vi "Oclaro_FB_INJ_RandomSampling.vi"(1 "Resistance (k Ohms)":dbl=10.0) -> ()   [LabVIEW 2014]
doc: "Use this template to measure or generate signals using the DAQ Assistant Express VI and NI-DAQmx. Double click the DAQ Assistant Express VI to launch a configuration wizard which steps you through configuring a measurement or generation.\n\nNote: You must have an NI-DAQmx compatible device installed to use this Express VI. Refer to the DAQ Quick Start Guide for NI-DAQ 7.0 for a list of compatible devices."
uses:
  Instance           8 18Saved   INJ FB Map .vi
  <instrlib>/Tektronix 7000 Series/Public/Data/Read (Single Waveform).vi
  <instrlib>/Tektronix 7000 Series/Tektronix 7000 Series.lvlib
  <userlib>/libbristoldlv/libbristoldlv.lvlib
  <userlib>/libbristoldlv/libbristoldlv.dll
panel:
  in  "Reset to 0 between settings?":bool
  out "Current Source":string="PROFILE-ITC510"
  out "Total Time (hrs)":dbl=23.33940424164136
  out "Finish time":timestamp=timestamp(3525397732.18738 s since 1904-01-01)
  out "Current INJ":dbl
  in  "file path":path=path "Z:/Toomey/Experimental Data/Oclaro/2015-09-18/Run01/Data"
  in  "Time Series Length":dbl=500000.0
  in  "OSA Model":string="Bristol-771"
  in  "Scope Model":string="Tektronix MSO 71254"
  in  "Exit":bool
  out "Iteration":i32
  out "Spectral Peak":dbl=0.8513913993644499 format="%#_10g"
  in  "Units":enum16{"GHz", "um", "cm-1"}(ring)=enum."um"
  in  "Max Wavelength (um)":ext=0.9
  in  "Min Wavelength (um)":ext=0.8
  out "Instrument Status:":string="OK"
  out "temperature":dbl=29.80661392211914
  out "pressure":dbl=779.7882080078125
  in  "Model":bool=TRUE
  in  "Channel (0: Channel 1)":u16(ring)=3 format="%#_5f" items=["Channel 1", "Channel 2", "Channel 3", "Channel 4", "Math 1", "Math 2", "Math 3", "Math 4", "Reference 1", "Reference 2", "Reference 3", "Reference 4"]
  out "Current AOM":dbl=0.9
  in  "Network Address":string="10.199.199.1"
  out "CL DLL Version":string="5.4.0"
  out "LV DLL Version":string="5.1.0"
  in  "Resolution":bool=TRUE
  in  "Select Wavelength Range":T1(ring)=enum."NIR II: 633 - 1700 nm"
  out "Error out":errorcluster
  in  "Capture OSA?":bool=TRUE
  in  "AOM Step":dbl=0.005
  in  "AOM Finish":dbl=0.9
  in  "AOM Start":dbl=0.1
  in  "Initial Current (mA)":dbl=15.0
  in  "Step Size (mA)":dbl=0.5
  in  "Max Current (mA)":dbl=85.0
  in  "AOM Channel":bool
  out "Start time":timestamp=timestamp(3523998390.26649 s since 1904-01-01)
  in  "Current Source Address":refnum<visa-resource-name>="GPIB0::3::INSTR"
  in  "TEC Address":refnum<visa-resource-name>="GPIB0::3::INSTR"
  in  "Tek Scope Address":refnum<visa-resource-name>="GPIB0::4::INSTR"
  in  "Time to wait for TEC (sec)":dbl=3.0 caption="Delay Time (s)"
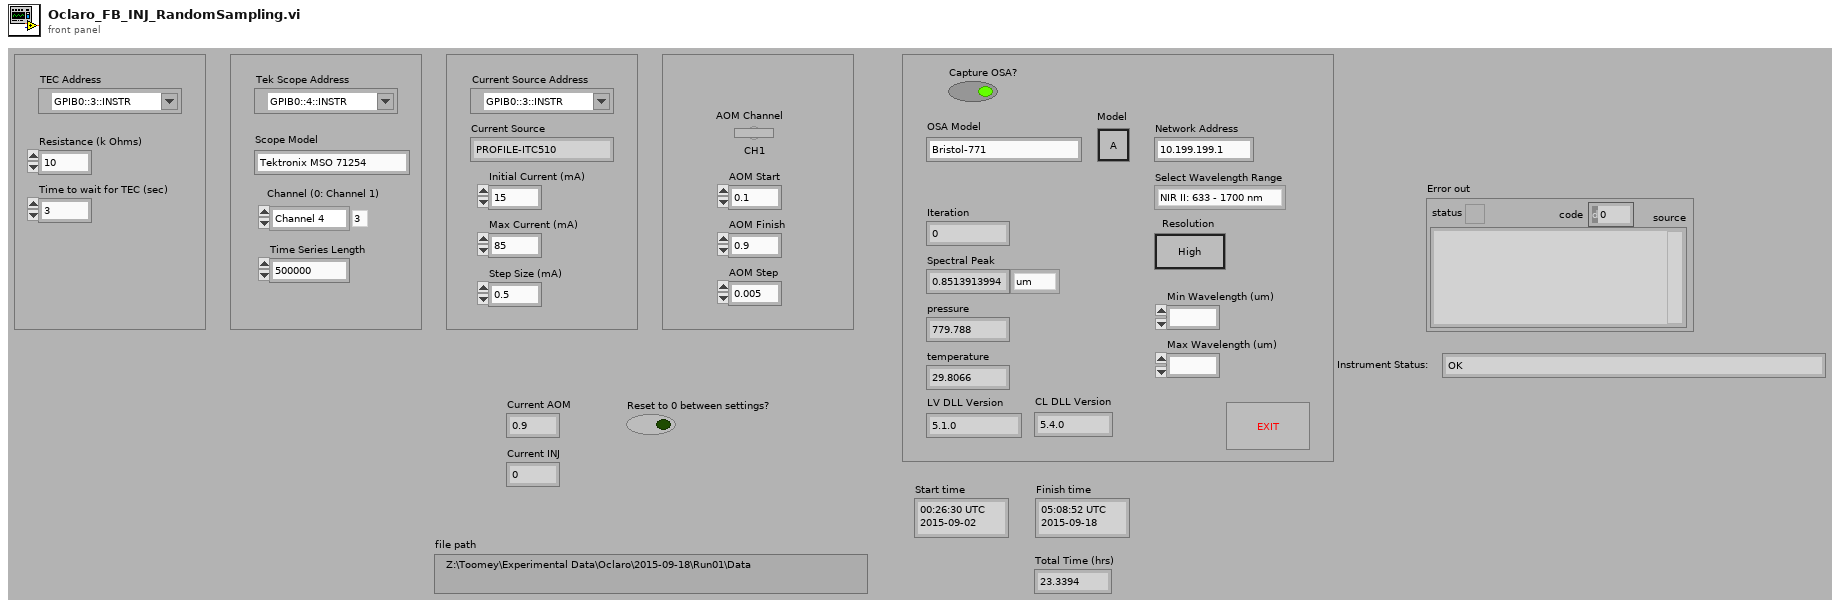
[diagram p1: front panel]
types:
  T1 = enum16{"VIS I: 375 - 633 nm", "VIS II: 633 - 1100 nm", "NIR I: 520 - 633 nm", "NIR II: 633 - 1700 nm", "IR: 1,000 - 5,000 nm", "MIR: 2,000 - 12,000 nm"}
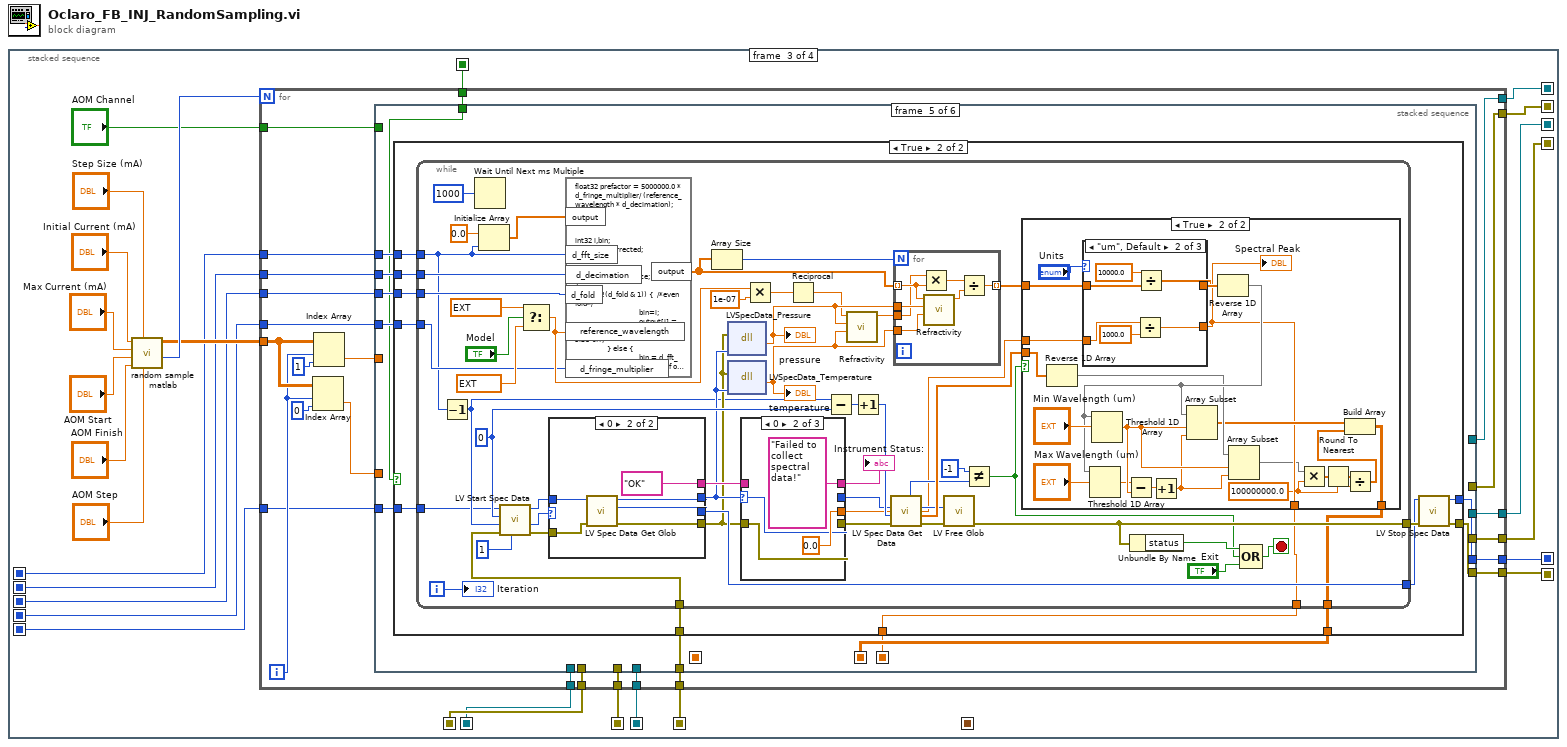
[diagram p0: block diagram]
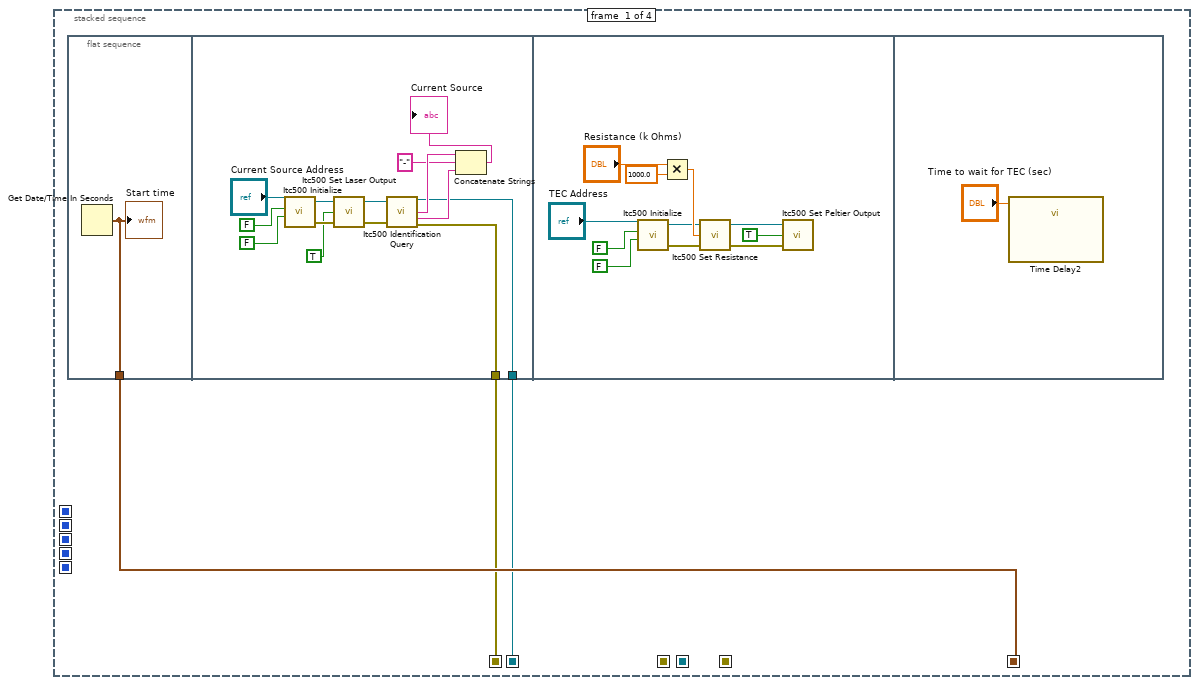
[diagram p2: hidden frame]
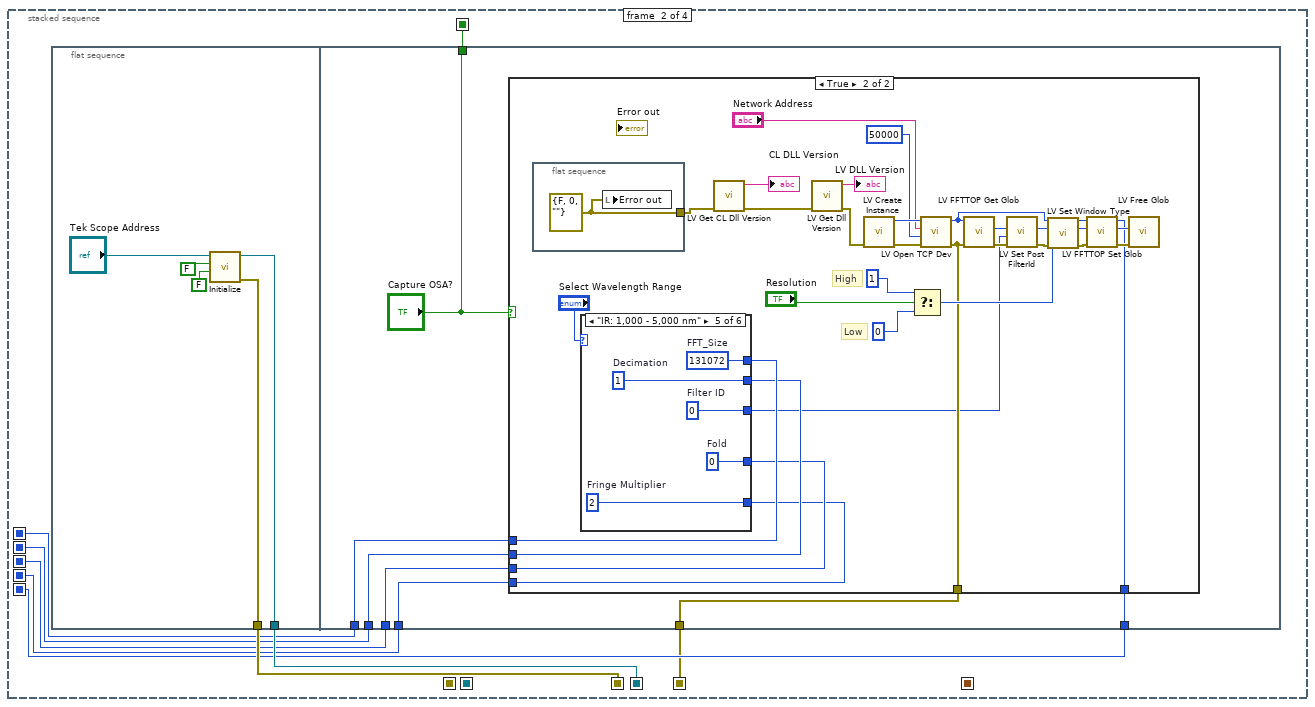
[diagram p3: hidden frame]
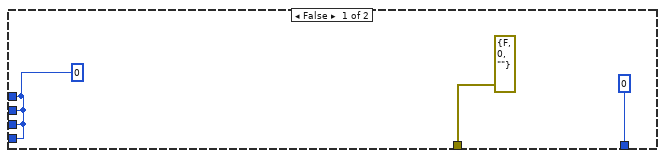
[diagram p4: hidden frame]
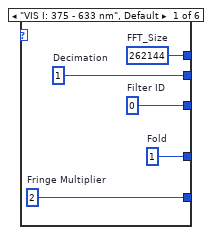
[diagram p5: hidden frame]
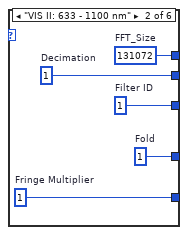
[diagram p6: hidden frame]
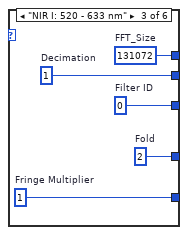
[diagram p7: hidden frame]
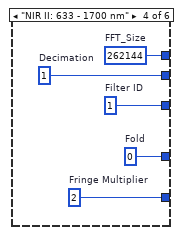
[diagram p8: hidden frame]
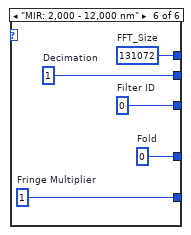
[diagram p9: hidden frame]
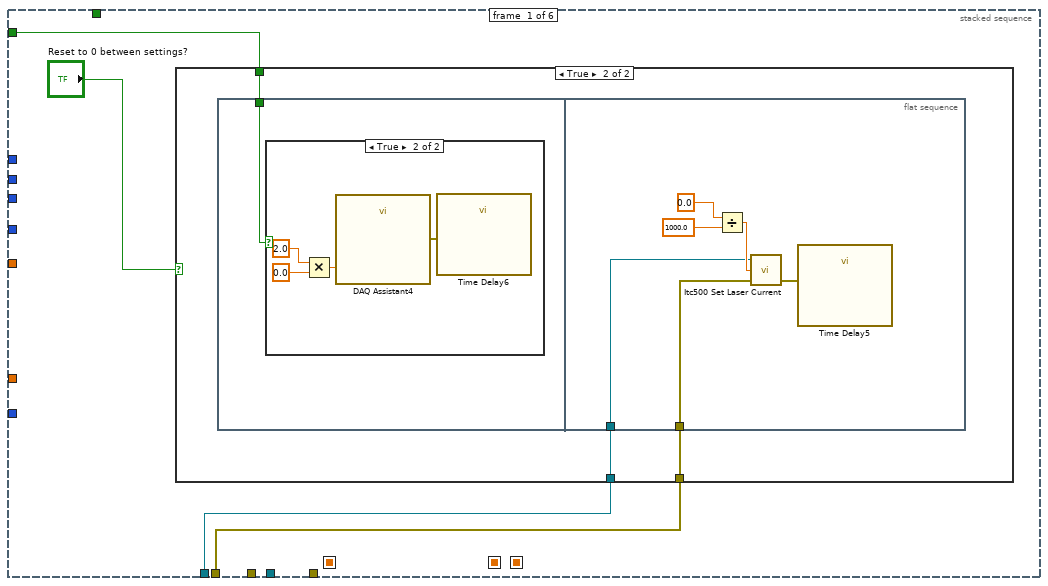
[diagram p10: hidden frame]
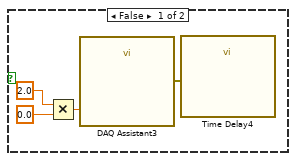
[diagram p12: hidden frame]
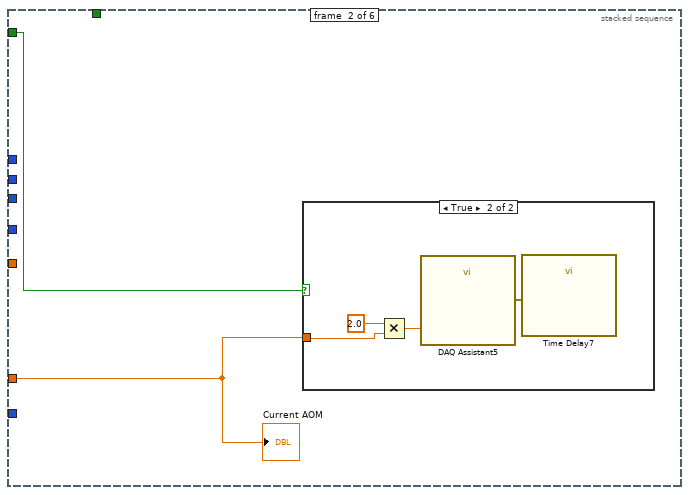
[diagram p13: hidden frame]
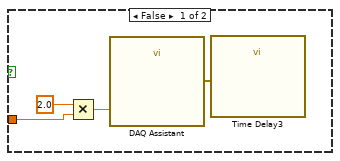
[diagram p14: hidden frame]
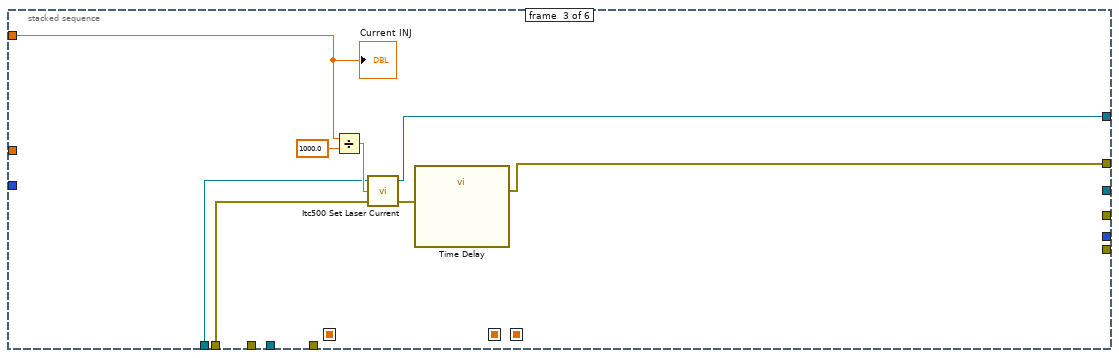
[diagram p15: hidden frame]
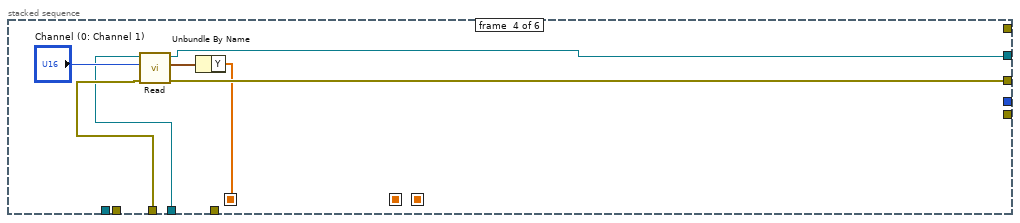
[diagram p16: hidden frame]
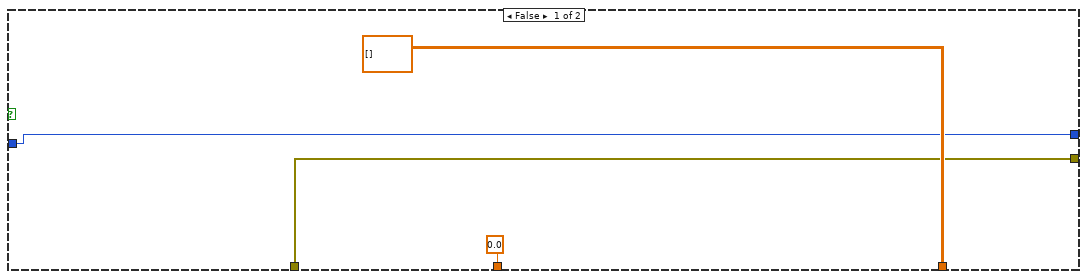
[diagram p17: hidden frame]
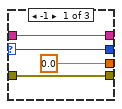
[diagram p18: hidden frame]
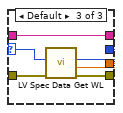
[diagram p19: hidden frame]
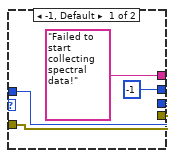
[diagram p20: hidden frame]
diagram:
  n1 = stacked-sequence {
    seq-local: [_ w38 _ _] -> [_ _ w121 _]
    seq-local: [_ w39 _ _] -> [_ _ w120 _]
    seq-local: [_ _ w122 _] -> [_ _ _ w383]
    seq-local: [_ _ w123 _] -> [_ _ _ w382]
    seq-local: [w3 _ _ _] -> [_ _ _ w384]
    seq-local: [_ _ w119 _] -> [_ _ _ w381]
    seq-local: [_ _ w118 _] -> [_ _ _ w380]
    seq-local: [w1 _ _ _] -> [_ _ w133 _]
    seq-local: [w2 _ _ _] -> [_ _ w134 _]
    seq-local: [_ w34 _ _] -> [_ _ w130 _]
    seq-local: [_ w35 _ _] -> [_ _ w129 _]
    seq-local: [_ w36 _ _] -> [_ _ w128 _]
    seq-local: [_ w37 _ _] -> [_ _ w127 _]
    seq-local: [_ w33 _ _] -> [_ _ w126 _]
    seq-local: [_ w32 _ _] -> [_ _ w125 _]
    seq-local: [_ w31 _ _] -> [_ _ w124 _]
    seq-local: [_ _ w117 _] -> [_ _ _ w379]
    seq-local: [_ _ w116 _] -> [_ _ _ w378]
    frame #0 {
      n2 = flat-sequence {
        tunnel: [w4] -> w3
        tunnel: [w7] -> w2
        tunnel: [w5] -> w1
        frame #0 {
          n3 = Get Date/Time In Seconds() -> (seconds since 1Jan1904=w4:timestamp)
          "Start time" <- w4
        }
        frame #1 {
          n4 = call <instrlib>:"Itc500 Initialize.vi"("reset device"=FALSE, "id query"=FALSE, "resource name"="Current Source Address") -> ("error out"=w18:errorcluster, "instrument handle"=w17:refnum<visa-resource-name>)  [unwired: 1 in, 1 out]
          n5 = call <instrlib>:"Itc500 Set Laser Output.vi"("error in (no error)"=w18, "output"=TRUE, "instrument handle"=w17) -> ("error out"=w8:errorcluster, "instrument handle out"=w6:refnum<visa-resource-name>)  [unwired: 1 out]
          n6 = call <instrlib>:"Itc500 Identification Query.vi"("instrument handle"=w6, "error in (no error)"=w8) -> ("instrument handle out"=w5:refnum<visa-resource-name>, "manufacturer name"=w12:string, "instrument name"=w11:string, "error out"=w7:errorcluster)  [unwired: 7 in, 3 out]
          n7 = Concatenate Strings(w12, "-" ("string"), w11) -> (→"Current Source":string)
        }
        frame #2 {
          n8 = call <instrlib>:"Itc500 Initialize.vi"("reset device"=FALSE, "id query"=FALSE, "resource name"="TEC Address") -> ("error out"=w25:errorcluster, "instrument handle"=w24:refnum<visa-resource-name>)  [unwired: 1 in, 1 out]
          n9 = Multiply(x="Resistance (k Ohms)", y=1000.0) -> (x*y=w28:dbl)
          n10 = call <instrlib>:"Itc500 Set Resistance.vi"("error in (no error)"=w25, "resistance"=w28, "instrument handle"=w24) -> ("error out"=w22:errorcluster, "instrument handle out"=w21:refnum<visa-resource-name>)  [unwired: 1 out]
          n11 = call <instrlib>:"Itc500 Set Peltier Output.vi"("error in (no error)"=w22, "output"=TRUE, "instrument handle"=w21) -> ()  [unwired: 3 out]
        }
        frame #3 {
          n12 = call "Time Delay2"("Delay Time (s)"="Time to wait for TEC (sec)") -> ()  [unwired: 10 in, 1 out]
        }
      }
    }
    frame #1 {
      n13 = flat-sequence {
        tunnel: [w41] -> w39
        tunnel: [w40] -> w38
        tunnel: [w51] -> w37
        tunnel: [w50] -> w36
        tunnel: [w49] -> w35
        tunnel: [w48] -> w34
        tunnel: ["Capture OSA?"] -> w33
        tunnel: [w46] -> w32
        tunnel: [w45] -> w31
        frame #0 {
          n14 = call <instrlib>:"Initialize.vi"("Reset? ( Yes)"=FALSE ("Reset (T: Reset)"), "ID Query? ( Yes)"=FALSE ("Reset (T: Reset)"), "VISA resource name"="Tek Scope Address") -> ("error out"=w40:errorcluster, "VISA resource name out"=w41:refnum<visa-resource-name>)  [unwired: 7 in]
        }
        frame #1 {
          n15 = case shown="True" "Capture OSA?" {
            tunnel: [errorcluster {"status"=FALSE, "code"=0, "source"=""} ("error out") w63] -> w45
            tunnel: [0 ("Handle out") w62] -> w46
            tunnel: [w52 w60] -> w48
            tunnel: [w52 w59] -> w49
            tunnel: [w52 w58] -> w50
            tunnel: [w52 w57] -> w51
            frame False {
              w52 = 0 ("FFT_Size")
            }
            frame True {
              # "High"
              # "Low"
              n16 = flat-sequence {
                tunnel: [w84] -> w56
                frame #0 {
                  w84 = errorcluster {"status"=FALSE, "code"=0, "source"=""} ("error out")
                  n17 = local write "Error out"(w84) -> ()
                }
              }
              n18 = case shown="\"IR: 1,000 - 5,000 nm\"" "Select Wavelength Range" {
                tunnel: [w89 w91 w96 w101 w106 w114] -> w57
                tunnel: [w88 w92 w97 w102 w107 w113] -> w58
                tunnel: [w87 w93 w98 w103 w108 w112] -> w59
                tunnel: [w86 w94 w99 w104 w109 w111] -> w60
                tunnel: [w85 w90 w95 w100 w105 w110] -> w55
                frame "VIS I: 375 - 633 nm", Default {
                  w85 = i8 0  # Filter ID
                  w89 = 2  # Fringe Multiplier
                  w88 = 1  # Fold
                  w87 = 1  # Decimation
                  w86 = 262144  # FFT_Size
                }
                frame "VIS II: 633 - 1100 nm" {
                  w90 = i8 1  # Filter ID
                  w91 = 1  # Fringe Multiplier
                  w92 = 1  # Fold
                  w93 = 1  # Decimation
                  w94 = 131072  # FFT_Size
                }
                frame "NIR I: 520 - 633 nm" {
                  w95 = i8 0  # Filter ID
                  w96 = 1  # Fringe Multiplier
                  w97 = 2  # Fold
                  w98 = 1  # Decimation
                  w99 = 131072  # FFT_Size
                }
                frame "NIR II: 633 - 1700 nm" {
                  w100 = i8 1  # Filter ID
                  w101 = 2  # Fringe Multiplier
                  w102 = 0  # Fold
                  w103 = 1  # Decimation
                  w104 = 262144  # FFT_Size
                }
                frame "IR: 1,000 - 5,000 nm" {
                  w105 = i8 0  # Filter ID
                  w106 = 2  # Fringe Multiplier
                  w107 = 0  # Fold
                  w108 = 1  # Decimation
                  w109 = 131072  # FFT_Size
                }
                frame "MIR: 2,000 - 12,000 nm" {
                  w110 = i8 0  # Filter ID
                  w114 = 1  # Fringe Multiplier
                  w113 = 0  # Fold
                  w112 = 1  # Decimation
                  w111 = 131072  # FFT_Size
                }
              }
              n19 = call <userlib>:"LV Get CL Dll Version.vi"("error in (no error)"=w56) -> ("error out"=w76:errorcluster, "str out"=→"CL DLL Version":string)  [unwired: 8 in]
              n20 = call <userlib>:"LV Get Dll Version.vi"("error in (no error)"=w76) -> ("error out"=w77:errorcluster, "str out"=→"LV DLL Version":string)  [unwired: 8 in]
              n21 = call <userlib>:"LV Create Instance.vi"("error in (no error)"=w77) -> ("error out"=w80:errorcluster, "function return (Handle)"=w83:i32)  [unwired: 9 in]
              n22 = Select(t=i8 1, s="Resolution", f=i8 0) -> (s? t:f=w64:i8)
              n23 = call <userlib>:"LV Open TCP Dev.vi"("error in (no error)"=w80, "Port"=u16 50000 ("IP Port"), "TCP/IP Address"="Network Address", "Handle in"=w83) -> ("error out"=w63:errorcluster, "Handle out"=w73:i32)  [unwired: 6 in]
              n24 = call <userlib>:"LV FFTTOP Get Glob.vi"("error in (no error)"=w63, "Handle in"=w73) -> ("error out"=w74:errorcluster, "GHandle out"=w75:i32)  [unwired: 7 in, 1 out]
              n25 = call <userlib>:"LV Set Post FilterId.vi"("error in (no error)"=w74, "Filter ID"=w55, "GHandle in"=w75) -> ("error out"=w69:errorcluster, "GHandle out"=w70:i32)  [unwired: 7 in]
              n26 = call <userlib>:"LV Set Window Type.vi"("error in (no error)"=w69, "Resolution"=w64, "GHandle in"=w70) -> ("error out"=w68:errorcluster)  [unwired: 5 in, 2 out]
              n27 = call <userlib>:"LV FFTTOP Set Glob.vi"("error in (no error)"=w68, "GHandle in"=w70, "Handle in"=w73) -> ("error out"=w71:errorcluster, "GHandle out"=w72:i32, "Handle out"=w62:i32)  [unwired: 6 in]
              n28 = call <userlib>:"LV Free Glob.vi"("error in (no error)"=w71, "GHandle in"=w72) -> ()  [unwired: 9 in, 1 out]
            }
          }
        }
      }
    }
    frame #2 {
      n29 = call "random sample matlab.vi"("AOM delta"="AOM Step", "INJ delta"="Step Size (mA)", "AOM end"="AOM Finish", "AOM start"="AOM Start", "INJ end"="Max Current (mA)", "INJ start"="Initial Current (mA)") -> ("No. of parameters"=w132:i32, "Shuffled Parameters"=w131:dbl[][])  [unwired: 4 in]
      n30 = for {
        N: w132 -> [_]
        tunnel: w134 -> [w164]
        tunnel: w133 -> [w163]
        tunnel: w131 -> [w161]
        tunnel: w130 -> [w156]
        tunnel: w129 -> [w155]
        tunnel: w128 -> [w154]
        tunnel: w127 -> [w153]
        tunnel: w126 -> [w152]
        tunnel: w125 -> [w151]
        tunnel: w124 -> [w150]
        tunnel: [w149] -> w123
        tunnel: [w148] -> w122
        tunnel: w121 -> [w147]
        tunnel: w120 -> [w146]
        tunnel: [w145] -> w119
        tunnel: [w144] -> w118
        tunnel: [w143] -> w117
        tunnel: [w142] -> w116
        tunnel: "AOM Channel" -> [w141]
        i -> [w160]
        n31 = Index Array(array=w161, index (row)=w160, index (col)=0 ("disabled index (col)")) -> (element=w157:dbl)
        n32 = Index Array(array=w161, index (row)=w160, index (col)=1 ("disabled index (col)")) -> (element=w158:dbl)
        n33 = stacked-sequence {
          seq-local: [_ _ _ w207 _ _] -> [_ _ _ _ _ w375]
          seq-local: [_ _ _ _ w222 _] -> [_ _ _ _ _ w364]
          seq-local: [_ _ _ _ w219 _] -> [_ _ _ _ _ w363]
          tunnel: [_ _ w199 _ _ _] -> w149
          tunnel: [_ _ _ w210 _ _] -> w145
          tunnel: [_ _ _ w208 _ _] -> w144
          tunnel: w164 -> [w167 _ w201 _ _ _]
          tunnel: w163 -> [w168 _ w200 _ _ _]
          tunnel: [_ _ w198 _ _ _] -> w148
          tunnel: [_ _ _ _ w221 _] -> w143
          tunnel: [_ _ _ _ w220 _] -> w142
          tunnel: w158 -> [_ _ w197 _ _ _]
          tunnel: w157 -> [_ w188 _ _ _ _]
          tunnel: w156 -> [_ _ _ _ w218 _]
          tunnel: w155 -> [_ _ _ _ w217 _]
          tunnel: w154 -> [_ _ _ _ w216 _]
          tunnel: w153 -> [_ _ _ _ w215 _]
          tunnel: w152 -> [_ _ _ _ w214 w362]
          tunnel: w151 -> [_ _ _ _ w213 _]
          tunnel: w150 -> [_ _ _ _ w212 _]
          tunnel: w147 -> [_ _ _ w206 _ _]
          tunnel: w146 -> [_ _ _ w205 _ _]
          tunnel: w141 -> [w165 w187 _ _ _ _]
          frame #0 {
            n34 = case shown="True" "Reset to 0 between settings?" {
              tunnel: w168 -> [_ w171]
              tunnel: w167 -> [_ w170]
              tunnel: w165 -> [_ w169]
              frame False {
              }
              frame True {
                n35 = flat-sequence {
                  tunnel: w169 -> [w172]
                  tunnel: w171 -> [w183]
                  tunnel: w170 -> [w182]
                  frame #0 {
                    n36 = case shown="True" w172 {
                      frame False {
                        n37 = Multiply(x=2.0, y=0.0 ("data")) -> (x*y=w173:dbl)
                        n38 = call "DAQ Assistant3"("data"=w173) -> ("error out"=w176:errorcluster)  [unwired: 17 in, 1 out]
                        n39 = call "Time Delay4"("error in (no error)"=w176) -> ()  [unwired: 10 in, 1 out]
                      }
                      frame True {
                        n40 = Multiply(x=2.0, y=0.0 ("data")) -> (x*y=w180:dbl)
                        n41 = call "DAQ Assistant4"("data"=w180) -> ("error out"=w177:errorcluster)  [unwired: 17 in, 1 out]
                        n42 = call "Time Delay6"("error in (no error)"=w177) -> ()  [unwired: 10 in, 1 out]
                      }
                    }
                  }
                  frame #1 {
                    n43 = Divide(x=0.0, y=1000.0) -> (x/y=w184:dbl)
                    n44 = call <instrlib>:"Itc500 Set Laser Current.vi"("error in (no error)"=w182, "current"=w184, "instrument handle"=w183) -> ("error out"=w185:errorcluster)  [unwired: 2 out]
                    n45 = call "Time Delay5"("error in (no error)"=w185) -> ()  [unwired: 10 in, 1 out]
                  }
                }
              }
            }
          }
          frame #1 {
            n46 = case shown="True" w187 {
              tunnel: w188 -> [w189 w193]
              frame False {
                n47 = Multiply(x=2.0, y=w189) -> (x*y=w192:dbl)
                n48 = call "DAQ Assistant"("data"=w192) -> ("error out"=w191:errorcluster)  [unwired: 17 in, 1 out]
                n49 = call "Time Delay3"("error in (no error)"=w191) -> ()  [unwired: 10 in, 1 out]
              }
              frame True {
                n50 = Multiply(x=2.0, y=w193) -> (x*y=w194:dbl)
                n51 = call "DAQ Assistant5"("data"=w194) -> ("error out"=w195:errorcluster)  [unwired: 17 in, 1 out]
                n52 = call "Time Delay7"("error in (no error)"=w195) -> ()  [unwired: 10 in, 1 out]
              }
            }
            "Current AOM" <- w188
          }
          frame #2 {
            n53 = Divide(x=w197, y=1000.0) -> (x/y=w202:dbl)
            n54 = call <instrlib>:"Itc500 Set Laser Current.vi"("error in (no error)"=w201, "current"=w202, "instrument handle"=w200) -> ("error out"=w203:errorcluster, "instrument handle out"=w198:refnum<visa-resource-name>)  [unwired: 1 out]
            n55 = call "Time Delay"("error in (no error)"=w203) -> ("error out"=w199:errorcluster)  [unwired: 10 in]
            "Current INJ" <- w197
          }
          frame #3 {
            n56 = call-poly <instrlib>:"Read.vi"("error in (no error)"=w206, "Channel (0: Channel 1)"="Channel (0: Channel 1)", "VISA resource name"=w205) -> ("error out"=w208:errorcluster, "Waveform Data"=w211:waveform(dbl), "VISA resource name out"=w210:refnum<visa-resource-name>)  [unwired: 6 in]
            n57 = Unbundle By Name(w211) -> ("Y"=w207:dbl[])
          }
          frame #4 {
            n58 = case shown="True" w214 {
              tunnel: [ext[][] [] w238] -> w222
              tunnel: [w224 w235] -> w221
              tunnel: [w223 w234] -> w220
              tunnel: [0.0 w233] -> w219
              tunnel: w218 -> [_ w232]
              tunnel: w217 -> [_ w231]
              tunnel: w216 -> [_ w230]
              tunnel: w215 -> [_ w229]
              tunnel: w213 -> [w224 w228]
              tunnel: w212 -> [w223 w227]
              frame False {
              }
              frame True {
                n59 = while {
                  tunnel: [w279] -> w237
                  tunnel: [w274] -> w236
                  tunnel: [w246] -> w238
                  tunnel: [w245] -> w233
                  tunnel: w232 -> [w239]
                  tunnel: w231 -> [w244]
                  tunnel: w230 -> [w243]
                  tunnel: w229 -> [w242]
                  tunnel: w228 -> [w241]
                  tunnel: w227 -> [w240]
                  i -> [w289]
                  stop <- w251 stop-if-true
                  w284 = 0 ("IP Port")
                  n60 = Decrement(x=w239) -> (x-1=w247:i32)
                  n61 = Wait Until Next ms Multiple(millisecond multiple=u32 1000) -> ()  [unwired: 1 out]
                  n62 = Initialize Array(0.0 ("output variable"), w239) -> (w264:dbl[])
                  n63 = call <userlib>:"LV Start Spec Data.vi"("Count"=1 ("IP Port"), "error in (no error)"=w240, "End Bin"=w247, "Start Bin"=w284, "Handle in"=w241) -> ("error out"=w275:errorcluster, "function return code"=w276:i32, "Handle out"=w281:i32)  [unwired: 3 in]
                  n64 = Select(t=ext 632.9914, s="Model", f=ext 632.991) -> (s? t:f=w252:ext)
                  n65 = case shown="0" w276 {
                    tunnel: w281 -> [w314 w320]
                    tunnel: [-1 ("IP Port") w319] -> w269
                    tunnel: [w314 w318] -> w274
                    tunnel: w275 -> [w313 w317]
                    tunnel: [w313 w316] -> w268
                    tunnel: ["Failed to start collecting spectral data!" "OK"] -> w272
                    frame -1, Default {
                    }
                    frame 0 {
                      n66 = call <userlib>:"LV Spec Data Get Glob.vi"("error in (no error)"=w317, "Handle in"=w320) -> ("error out"=w316:errorcluster, "GHandle out"=w319:i32, "Handle out"=w318:i32)  [unwired: 7 in]
                    }
                  }
                  n67 = formula code="float32 prefactor = 5000000.0 * d_fringe_multiplier/ (reference_wavelength * d_decimation);\n\n\n\nint32 i,bin;\nfloat32 uncorrected;\n\n                \nfor(i = 0; i<d_fft_size; i++)\n{\n         if (!(d_fold & 1)) {  /*even fold*/\n                                bin=i;\n                                output[i] = prefactor * (d_fold + bin/(d_fft_size-0));\n                } else {\n                                bin = d_fft_size - i - 1; /*reverse array if odd fold*/\n                                output[i] = prefactor * (d_fold + 1.0 - bin/d_fft_size);\n                }\n                  \n}"("d_fft_size"=w239, "d_decimation"=w244, "d_fold"=w243, "d_fringe_multiplier"=w242, "output"=w264, "reference_wavelength"=w252) -> ("output"=w259:dbl[])
                  n68 = Array Size(array=w259) -> (size(s)=w267:i32)
                  n69 = dll-call lib="C:/Program Files (x86)/National Instruments/LabVIEW 2014/user.lib/libbristoldlv/libbristoldlv.dll" fn="LVSpecData_Pressure"(error in=w268, "ghandle"=w269) -> ("pressure"=w263:dbl)  [unwired: 3 in, 2 out]
                  "pressure" <- w263
                  n70 = dll-call lib="C:/Program Files (x86)/National Instruments/LabVIEW 2014/user.lib/libbristoldlv/libbristoldlv.dll" fn="LVSpecData_Temperature"(error in=w268, "ghandle"=w269) -> ("temperature"=w262:dbl)  [unwired: 3 in, 2 out]
                  "temperature" <- w262
                  n71 = case shown="0" w269 {
                    selector: w269 -> [w299 w303 w308]
                    tunnel: [0.0 ("IP Port") 0.0 ("IP Port") w310] -> w260
                    tunnel: w268 -> [w298 w302 w309]
                    tunnel: [w299 w303 w307] -> w271
                    tunnel: [w298 w302 w306] -> w273
                    tunnel: [w300 "Failed to collect spectral data!" w305] -> w270
                    tunnel: w272 -> [w300 _ w305]
                    frame -1 {
                    }
                    frame 0 {
                    }
                    frame Default {
                      n72 = call <userlib>:"LV Spec Data Get WL.vi"("GHandle in"=w308, "error in (no error)"=w309) -> ("GHandle out"=w307:i32, "Wavelength"=w310:dbl, "error out"=w306:errorcluster)  [unwired: 6 in]
                    }
                  }
                  "Instrument Status:" <- w270
                  n73 = Multiply(x=w252, y=1e-07) -> (x*y=w255:ext)
                  n74 = Reciprocal(x=w255) -> (1/x=w253:ext)
                  n75 = Subtract(x=w247, y=w284) -> (x-y=w283:i32)
                  n76 = call "Refractivity.vi"("Temp"=w262, "Press"=w263, "Wavelength"=w253) -> ("Index [i]"=w266:ext)  [unwired: 8 in]
                  n77 = Increment(x=w283) -> (x+1=w282:i32)
                  n78 = call <userlib>:"LV Spec Data Get Data.vi"("error in (no error)"=w273, "max len"=w282, "GHandle in"=w271) -> ("error out"=w280:errorcluster, "Spectral Data"=w287:sgl[], "GHandle out"=w285:i32, "function return code"=w278:i32)  [unwired: 4 in]
                  n79 = for {
                    N: w267 -> [_]
                    tunnel: w259 -> [w292] mode=indexing
                    tunnel: [w293] -> w261 mode=indexing
                    tunnel: w263 -> [w296]
                    tunnel: w262 -> [w295]
                    tunnel: w266 -> [w291]
                    n80 = Multiply(x=w291, y=w292) -> (x*y=w294:ext)
                    n81 = call "Refractivity.vi"("Temp"=w295, "Press"=w296, "Wavelength"=w292) -> ("Index [i]"=w290:ext)  [unwired: 8 in]
                    n82 = Divide(x=w294, y=w290) -> (x/y=w293:ext)
                  }
                  n83 = call <userlib>:"LV Free Glob.vi"("error in (no error)"=w280, "GHandle in"=w285) -> ("error out"=w279:errorcluster)  [unwired: 9 in]
                  n84 = Not Equal?(x=-1, y=w278) -> (x != y?=w248:bool)
                  n85 = case shown="True" w248 {
                    tunnel: w287 -> [_ w339]
                    tunnel: w261 -> [_ w343]
                    tunnel: w260 -> [_ w341]
                    tunnel: [ext[][] [] w329] -> w246
                    tunnel: [0.0 w328] -> w245
                    frame False {
                    }
                    frame True {
                      w325 = 100000000.0 ("y")
                      n86 = Reverse 1D Array(array=w339) -> (reversed array=w334:sgl[])
                      n87 = case shown="\"um\", Default" "Units" {
                        tunnel: w343 -> [w349 w355 w360]
                        tunnel: [w347 w354 w360] -> w340
                        tunnel: w341 -> [w344 w352 w359]
                        tunnel: [w346 w351 w357] -> w328
                        frame "GHz" {
                          n88 = Divide(x=299792458.0, y=w344) -> (x/y=w346:dbl)
                          n89 = Multiply(x=w349, y=29.9792458) -> (x*y=w347:ext[])
                        }
                        frame "um", Default {
                          n90 = Divide(x=w352, y=1000.0) -> (x/y=w351:dbl)
                          n91 = Divide(x=10000.0, y=w355) -> (x/y=w354:ext[])
                        }
                        frame "cm-1" {
                          n92 = Multiply(x=w359, y=1e-07) -> (x*y=w358:dbl)
                          n93 = Reciprocal(x=w358) -> (1/x=w357:dbl)
                        }
                      }
                      "Spectral Peak" <- w328
                      n94 = Reverse 1D Array(array=w340) -> (reversed array=w336:ext[])
                      n95 = Threshold 1D Array(2:"Max Wavelength (um)", 3:w336) -> (0:w332:ext)  [unwired: 1 in]
                      n96 = Threshold 1D Array(2:"Min Wavelength (um)", 3:w336) -> (0:w335:ext)  [unwired: 1 in]
                      n97 = Subtract(x=w332, y=w335) -> (x-y=w331:ext)
                      n98 = Increment(x=w331) -> (x+1=w330:ext)
                      n99 = Array Subset(array=w336, index=w335, length=w330) -> (w333:ext[])
                      n100 = Array Subset(array=w334, index=w335, length=w330) -> (w324:sgl[])
                      n101 = Multiply(x=w324, y=w325) -> (x*y=w327:dbl[])
                      n102 = Round To Nearest(number=w327) -> (nearest integer value=w326:dbl[])
                      n103 = Divide(x=w326, y=w325) -> (x/y=w323:dbl[])
                      n104 = Build Array(w333, w323) -> (w329:ext[][])
                    }
                  }
                  n105 = Unbundle By Name(w279) -> ("status"=w250:bool)
                  n106 = Compound Arithmetic op=OR(w250, w248, "Exit") -> (w251:bool)
                  "Iteration" <- w289
                }
                n107 = call <userlib>:"LV Stop Spec Data.vi"("error in (no error)"=w237, "Handle in"=w236) -> ("error out"=w234:errorcluster, "Handle out"=w235:i32)  [unwired: 8 in]
              }
            }
          }
          frame #5 {
            n108 = local read "Current AOM"() -> (w366:dbl)
            n109 = local read "Current INJ"() -> (w361:dbl)
            n110 = local read "Current Source"() -> (w369:string)
            n111 = Path To String(path="file path") -> (string=w377:string)
            n112 = Boolean To (0,1)(Boolean=w362) -> (0, 1=w365:i16)
            n113 = Format Into String(format string="%05.2f", w361) -> (resulting string=w373:string)  [unwired: 2 in, 1 out]
            n114 = Format Into String(format string="%05.3f", w366) -> (resulting string=w374:string)  [unwired: 2 in, 1 out]
            n115 = script code="h5create([file_loc '/INJ_' INJval 'mA_AOM_' FBval 'V.h5'],'/TS',[1 TSlength],'ChunkSize',[1 TSlength],'Deflate',5)\n\nh5writeatt([file_loc '/INJ_' INJval 'mA_AOM_' FBval 'V.h5'],'/','var1',inj);\nh5writeatt([file_loc '/INJ_' INJval 'mA_AOM_' FBval 'V.h5'],'/','var1_name','Injection Current (mA)');\nh5writeatt([file_loc '/INJ_' INJval 'mA_AOM_' FBval 'V.h5'],'/','var2',fb);\nh5writeatt([file_loc '/INJ_' INJval 'mA_AOM_' FBval 'V.h5'],'/','var2_name','AOM_Voltage (V)');\nh5writeatt([file_loc '/INJ_' INJval 'mA_AOM_' FBval 'V.h5'],'/','Current_Source',current);\nh5writeatt([file_loc '/INJ_' INJval 'mA_AOM_' FBval 'V.h5'],'/','Temperature','25C');\n\nh5write([file_loc '/INJ_' INJval 'mA_AOM_' FBval 'V.h5'],'/TS',TSdata,[1 1],size(TSdata));\n\nh5writeatt([file_loc '/INJ_' INJval 'mA_AOM_' FBval 'V.h5'],'/TS','Oscilloscope_model',scope);\nh5writeatt([file_loc '/INJ_' INJval 'mA_AOM_' FBval 'V.h5'],'/TS','Sample_interval',20e-12);\nh5writeatt([file_loc '/INJ_' INJval 'mA_AOM_' FBval 'V.h5'],'/TS','Vertical_Scale','10mV/div');\nh5writeatt([file_loc '/INJ_' INJval 'mA_AOM_' FBval 'V.h5'],'/TS','Acquisition_Mode','Sample');\nh5writeatt([file_loc '/INJ_' INJval 'mA_AOM_' FBval 'V.h5'],'/TS','Sampling_Mode','Real-time');\n\nif spec == 1\nsize(OSAdata)\nh5create([file_loc '/INJ_' INJval 'mA_AOM_' FBval 'V.h5'],'/OSA',size(OSAdata),'ChunkSize',[1 length(OSAdata)],'Deflate',5)\nh5write([file_loc '/INJ_' INJval 'mA_AOM_' FBval 'V.h5'],'/OSA',OSAdata,[1 1],size(OSAdata));\nh5writeatt([file_loc '/INJ_' INJval 'mA_AOM_' FBval 'V.h5'],'/OSA','OSA_model',osa);\nh5writeatt([file_loc '/INJ_' INJval 'mA_AOM_' FBval 'V.h5'],'/OSA','Resolution','High');\nh5writeatt([file_loc '/INJ_' INJval 'mA_AOM_' FBval 'V.h5'],'/OSA','Wavelength_Peak',wP);\nend"("file_loc"=w377, "INJval"=w373, "FBval"=w374, "TSlength"="Time Series Length", "TSdata"=w375, "OSAdata"=w364, "inj"=w361, "fb"=w366, "current"=w369, "scope"="Scope Model", "osa"="OSA Model", "spec"=w365, "wP"=w363) -> ()  [unwired: 1 in, 1 out]
          }
        }
      }
    }
    frame #3 {
      n116 = flat-sequence {
        tunnel: w383 -> [w386]
        tunnel: w382 -> [w385]
        tunnel: w381 -> [w393]
        tunnel: w380 -> [w392]
        tunnel: w384 -> [w395]
        tunnel: w379 -> [w411]
        tunnel: w378 -> [w410]
        frame #0 {
          n117 = call <instrlib>:"Itc500 Set Laser Current.vi"("error in (no error)"=w385, "current"=0.0, "instrument handle"=w386) -> ("error out"=w389:errorcluster, "instrument handle out"=w388:refnum<visa-resource-name>)  [unwired: 1 out]
          n118 = call <instrlib>:"Itc500 Set Laser Output.vi"("error in (no error)"=w389, "output"=FALSE, "instrument handle"=w388) -> ()  [unwired: 3 out]
        }
        frame #1 {
          n119 = call "DAQ Assistant2"("data"=0.0) -> ()  [unwired: 17 in, 2 out]
        }
        frame #2 {
          n120 = call <instrlib>:"Close.vi"("error in (no error)"=w392, "VISA resource name"=w393) -> ()  [unwired: 9 in, 1 out]
        }
        frame #3 {
          n121 = Get Date/Time In Seconds() -> (seconds since 1Jan1904=w404:timestamp)
          "Finish time" <- w404
          n122 = local read "file path"() -> (w394:path)
          n123 = Format Date/Time String(seconds (now)=w395) -> (date/time string=w405:string)  [unwired: 2 in]
          n124 = Subtract(x=w404, y=w395) -> (x-y=w408:dbl)
          n125 = Divide(x=w408, y=3600.0) -> (x/y=→"Total Time (hrs)":dbl)
          n126 = Path To String(path=w394) -> (string=w397:string)
          n127 = Concatenate Strings(w397, "\\info.txt" ("string")) -> (w399:string)
          n128 = Format Date/Time String(seconds (now)=w404) -> (date/time string=w401:string)  [unwired: 2 in]
          n129 = String To Path(string=w399) -> (path=w398:path)
          n130 = Concatenate Strings("Start time = ", w405, "\r", "Finish time = ", w401) -> (w400:string)
          n131 = Write to Text File(file (use dialog)=w398, text=w400) -> ()  [unwired: 2 in, 3 out]
        }
        frame #4 {
          n132 = call <userlib>:"LV Destroy Instance.vi"("error in (no error)"=w410, "Handle in"=w411) -> ()  [unwired: 8 in, 2 out]
        }
      }
    }
  }
